vi "环形布尔.vi"() -> ()   [LabVIEW 2018]
panel:
  in  "等待时间（毫秒）":u32=500
  out "簇 2":T1
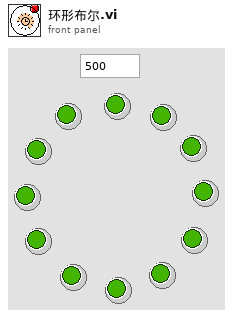
[diagram p1: front panel]
types:
  T1 = cluster{"布尔1":bool, "布尔 2":bool, "布尔 3":bool, "布尔 4":bool, "布尔 5":bool, "布尔 6":bool, "布尔 7":bool, "布尔 8":bool, "布尔 9":bool, "布尔 10":bool, "布尔 11":bool, "布尔 12":bool}
  T2 = cluster{"[0]":bool, "[1]":bool, "[2]":bool, "[3]":bool, "[4]":bool, "[5]":bool, "[6]":bool, "[7]":bool, "[8]":bool, "[9]":bool, "[10]":bool, "[11]":bool}
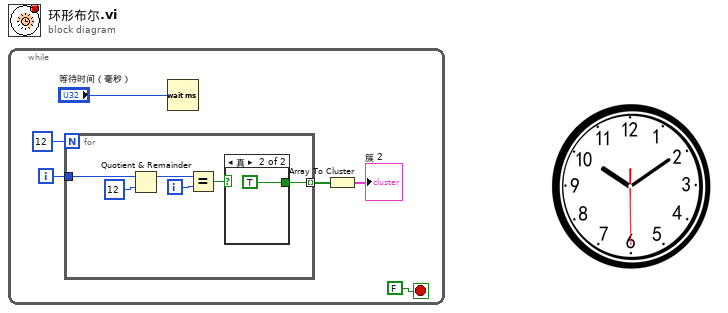
[diagram p0: block diagram]
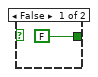
[diagram p2: hidden frame]
diagram:
  n1 = while {
    i -> [w4]
    stop <- FALSE stop-if-true
    n2 = for {
      N: 12 -> [_]
      tunnel: w4 -> [w9]
      tunnel: [w10] -> w2 mode=indexing
      i -> [w11]
      n3 = Quotient & Remainder(x=w9, y=12) -> (x-y*floor(x/y)=w7:i32)  [unwired: 1 out]
      n4 = Equal?(x=w7, y=w11) -> (x = y?=w12:bool)
      n5 = case shown="真" w12 {
        tunnel: [FALSE TRUE] -> w10
        frame False {
        }
        frame True {
        }
      }
    }
    n6 = Wait (ms)(milliseconds to wait="等待时间（毫秒）") -> ()  [unwired: 1 out]
    n7 = Array To Cluster(array=w2) -> (cluster=→"簇 2":T2)
  }
